vi "parse_syncChFixedSize.vi"(8 "error in (no error)":errorcluster, 9 "ChannelInfo":T2, 10 "AcquisitionStart":T4, 11 "Package String":string) -> (0 "error out":errorcluster, 1 "Timebase Frequency":dbl, 2 "Timestamp":dbl, 3 "Data":T1)   [LabVIEW 2020, in "OXYGEN_Datastream.lvlib"]
uses:
  OXYGEN_Datastream.lvlib
  TypeDefs/AcqInfo_AcquisitionStart.ctl
  TypeDefs/AcqInfo_AcquisitionStart_nanoseconds.ctl
  TypeDefs/ChannelInfo.ctl
  TypeDefs/ChannelInfo_Scaling.ctl
  TypeDefs/DataPoint_Variant.ctl
  parse_dataString.vi
panel:
  # "= (pckg size - 32) / 3"
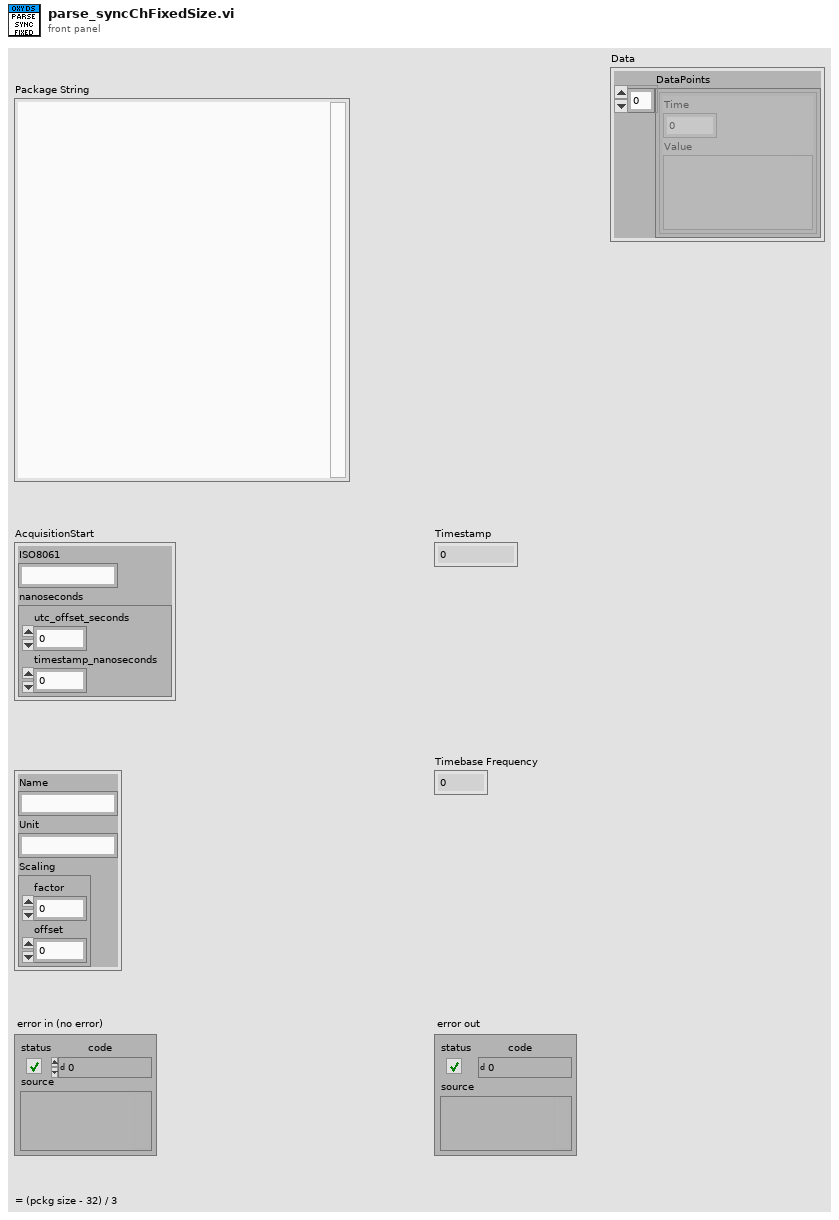
[diagram p1: front panel]
types:
  T1 = typedef "OXYGEN_Datastream.lvlib/DataPoint_Variant.ctl" = cluster{"DataPoints":cluster{"Time":dbl, "Value":variant}[]}
  T2 = typedef "OXYGEN_Datastream.lvlib/ChannelInfo.ctl" = cluster{"Name":string, "Unit":string, "Scaling":T3}
  T3 = typedef "OXYGEN_Datastream.lvlib/ChannelInfo_Scaling.ctl" = cluster{"factor":dbl, "offset":dbl}
  T4 = typedef "OXYGEN_Datastream.lvlib/AcqInfo_AcquisitionStart.ctl" = cluster{"ISO8061":string, "nanoseconds":T5}
  T5 = typedef "OXYGEN_Datastream.lvlib/AcqInfo_AcquisitionStart_nanoseconds.ctl" = cluster{"utc_offset_seconds":i64, "timestamp_nanoseconds":i64}
  T6 = enum16{"big-endian, network order", "native, host order", "little-endian"}
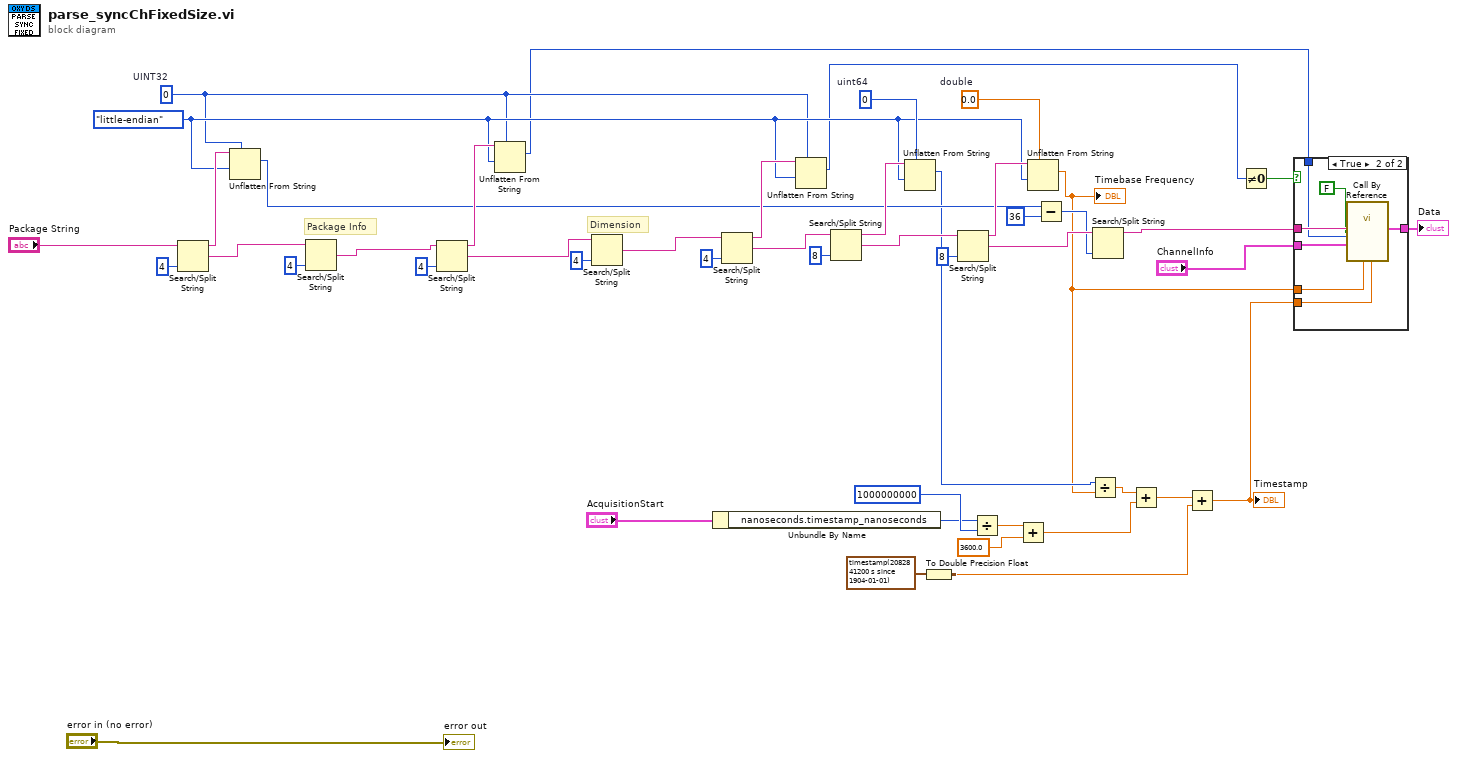
[diagram p0: block diagram]
diagram:
  w31 = 0.0  # double
  w34 = u64 0  # uint64
  w20 = u32 0  # UINT32
  w21 = T6."little-endian" ("byte order (0:big-endian, network order)")
  # "Package Info"
  # "Dimension"
  n1 = Search/Split String(string="Package String", offset (0)=4) -> (substring before match=w41:string, match + rest of string=w23:string)  [unwired: 1 in, 1 out]
  n2 = Unflatten From String(type=w20, binary string=w41, byte order (0:big-endian, network order)=w21) -> (value=w28:u32)  [unwired: 2 in, 2 out]
  n3 = Search/Split String(string=w23, offset (0)=4) -> (match + rest of string=w22:string)  [unwired: 1 in, 2 out]
  n4 = Search/Split String(string=w22, offset (0)=4) -> (substring before match=w39:string, match + rest of string=w42:string)  [unwired: 1 in, 1 out]
  n5 = Unflatten From String(type=w20, binary string=w39, byte order (0:big-endian, network order)=w21) -> (value=w18:u32)  [unwired: 2 in, 2 out]
  n6 = Search/Split String(string=w42, offset (0)=4) -> (match + rest of string=w40:string)  [unwired: 1 in, 2 out]
  n7 = Unbundle By Name("AcquisitionStart") -> ("nanoseconds.timestamp_nanoseconds"=w16:i64)
  n8 = Search/Split String(string=w40, offset (0)=4) -> (substring before match=w38:string, match + rest of string=w36:string)  [unwired: 1 in, 1 out]
  n9 = Unflatten From String(type=w20, binary string=w38, byte order (0:big-endian, network order)=w21) -> (value=w5:u32)  [unwired: 2 in, 2 out]
  n10 = Search/Split String(string=w36, offset (0)=8) -> (substring before match=w35:string, match + rest of string=w32:string)  [unwired: 1 in, 1 out]
  n11 = Unflatten From String(type=w34, binary string=w35, byte order (0:big-endian, network order)=w21) -> (value=w10:u64)  [unwired: 2 in, 2 out]
  n12 = To Double Precision Float(number=timestamp(2082841200 s since 1904-01-01)) -> (double precision float=w12:dbl)
  n13 = Search/Split String(string=w32, offset (0)=8) -> (substring before match=w30:string, match + rest of string=w29:string)  [unwired: 1 in, 1 out]
  n14 = Divide(x=w16, y=i64 1000000000) -> (x/y=w9:dbl)
  n15 = Add(x=w9, y=3600.0) -> (x+y=w8:dbl)
  n16 = Unflatten From String(type=w31, binary string=w30, byte order (0:big-endian, network order)=w21) -> (value=w3:dbl)  [unwired: 2 in, 2 out]
  "Timebase Frequency" <- w3
  n17 = Subtract(x=w28, y=u32 36) -> (x-y=w26:u32)
  n18 = Divide(x=w10, y=w3) -> (x/y=w14:dbl)
  n19 = Search/Split String(string=w29, offset (0)=w26) -> (substring before match=w19:string)  [unwired: 1 in, 2 out]
  n20 = Add(x=w14, y=w8) -> (x+y=w13:dbl)
  n21 = Add(x=w13, y=w12) -> (x+y=w4:dbl)
  "Timestamp" <- w4
  n22 = Not Equal To 0?(x=w5) -> (x != 0?=w6:bool)
  n23 = case shown="True" w6 {
    tunnel: w19 -> [_ w54]
    tunnel: w18 -> [_ w53]
    tunnel: "ChannelInfo" -> [_ w52]
    tunnel: w4 -> [_ w48]
    tunnel: w3 -> [_ w49]
    tunnel: [_ w51] -> w2
    frame False {
    }
    frame True {
      n24 = call-by-ref "?"("Timestamp"=w48, "Timebase Frequency"=w49, "Includes Timestamp?"=FALSE, "ChannelInfo"=w52, "Data Type"=w53, "Data String"=w54) -> ("Data"=w51:T1)  [unwired: 6 in, 3 out]
    }
  }
  "Data" <- w2
  "error out" <- "error in (no error)"
